vi "Repo Test.vi"   [LabVIEW 2019]
panel:
  # "test"
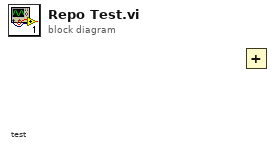
[diagram p0: block diagram]
diagram:
  # "test"
  n1 = Add() -> ()  [unwired: 2 in, 1 out]
